vi "Limelight Position.vi"(4 "Boolean":bool, 6 "Allowed Error":dbl, 7 "output range in":cluster{"output high":dbl, "output low":dbl}={"output high"=0.6, "output low"=-0.6} {"output low" format="%.2f"; "output high" format="%.2f"}, 9 "i Zone":dbl format="%.2f", 10 "PIDF gains":cluster{"Kp":dbl, "Ki":dbl, "Kd":dbl, "Kf":dbl}={"Kp"=0.06, "Ki"=0.0, "Kd"=0.0, "Kf"=0.0} {"Kf" format="%.3f"; "Kd" format="%.3f"; "Ki" format="%.3f"; "Kp" format="%.3f"}, 11 "Left Setpoint":dbl) -> (1 "Process Variable Vs. Setpoint":cluster{dbl, "setpoint":dbl}(graph), 2 "Right Motor Value":dbl, 3 "Left Motor Value":dbl, 5 "Left and Right Motor Values":T1(graph))   [LabVIEW 2018]
uses:
  <vilib>/Rock Robotics/Network Tables/NT Read Number.vi
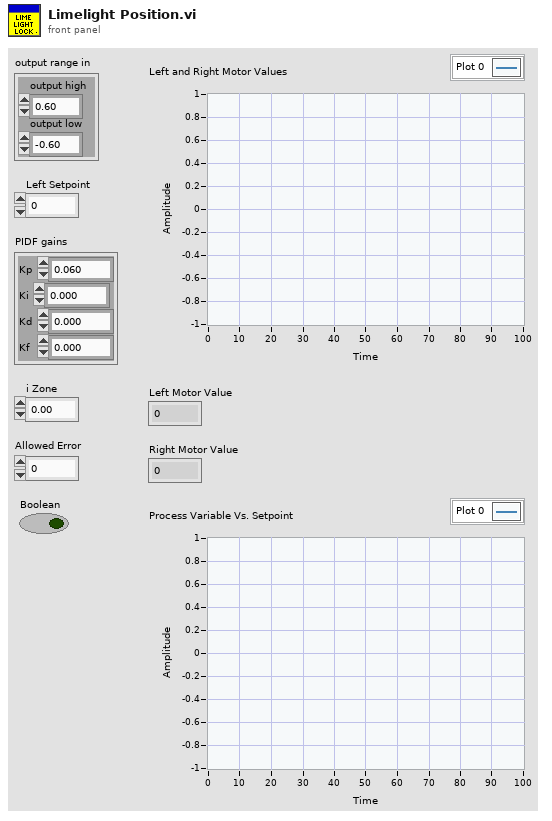
[diagram p1: front panel]
types:
  T1 = cluster{"Left Motor Value":dbl, "Right Motor Value":dbl}
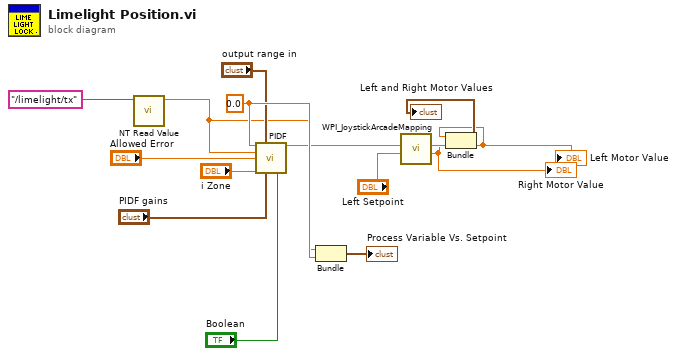
[diagram p0: block diagram]
diagram:
  w12 = 0.0 ("setpoint")
  n1 = call-poly <vilib>:"NT Read Value.vi"("Name"="/limelight/tx") -> ("Numeric"=w1:dbl)  [unwired: 9 in, 1 out]
  n2 = call "PIDF.vi"("setpoint"=w12, "output range"="output range in", "process variable"=w1, "Allowed Error"="Allowed Error", "i Zone"="i Zone", "PIDF gains"="PIDF gains", "reinitialize? (F)"="Boolean") -> ("output"=w8:dbl)  [unwired: 6 in, 2 out]
  n3 = Bundle("Numeric"=w1, "setpoint"=w12) -> (→"Process Variable Vs. Setpoint":cluster{"Numeric":dbl, "setpoint":dbl})  [unwired: 1 in]
  n4 = call <vilib>:"WPI_JoystickArcadeMapping.vi"("Y axis value"="Left Setpoint", "X axis value"=w8) -> ("Right Motor Value"=w2:dbl, "Left Motor Value"=w3:dbl)  [unwired: 8 in]
  "Right Motor Value" <- w2
  "Left Motor Value" <- w3
  n5 = Bundle("Left Motor Value"=w3, "Right Motor Value"=w2) -> (→"Left and Right Motor Values":T1)  [unwired: 1 in]
